vi "Main.vi"(8 "error in":errorcluster, 11 "Philosopher in":refnum<class "Philosopher.lvclass">) -> (0 "error out":errorcluster, 3 "Philosopher out":refnum<class "Philosopher.lvclass">)   [LabVIEW 2023, in "Philosopher.lvclass"]
uses:
  Philosopher.lvclass
  C:/Program Files (x86)/National Instruments/LabVIEW 2023/vi.lib/addons/_Workers/Library/Classes/Worker/Worker.lvclass
  Initialization Data.ctl
  <vilib>/addons/_Workers/Library/Classes/Message Queue/Message Queue.lvclass
  Philosopher.lvclass/Philosopher.ctl
  <vilib>/Utility/miscctls.llb/LVRectTypeDef.ctl
  <vilib>/addons/_Workers/Library/Classes/Message/Enqueue Message to Queue.vi
  <vilib>/addons/_Workers/Library/Classes/Message/Message.lvclass
  Table/Table.lvclass
  <vilib>/addons/_Workers/Library/Classes/Callback Message/Callback Message.lvclass
  Message Pump/Message Pump.lvclass
  <userlib>/_Workers/Worker Library/Message Pump/Workers/Message Pump/_Message Pump.lvclass
  C:/Program Files (x86)/National Instruments/LabVIEW 2023/vi.lib/addons/_Workers/Library/Classes/Workers Object/Workers Object.lvclass
  C:/Projects/DPP Workers/Workers/Philosopher/Philosopher.lvclass
panel:
  out "ID":i32
  out "State Picture":u16(ring)
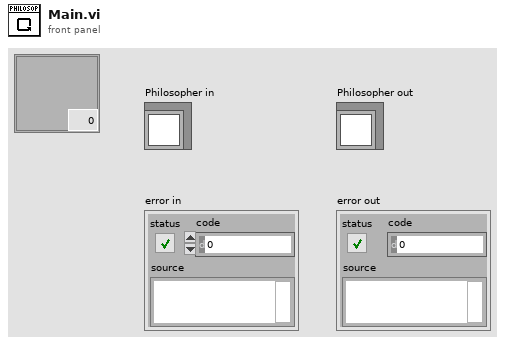
[diagram p1: front panel]
types:
  T1 = typedef "Philosopher.lvclass/Initialization Data.ctl" = cluster{"ID":i32, "MGQ Table":refnum<class "Message Queue.lvclass">}
  T2 = typedef "LVRectTypeDef.ctl" = cluster{"Left":i16, "Top":i16, "Right":i16, "Bottom":i16}
  T3 = typedef "Workers.lvlib/Case Label.ctl" = string
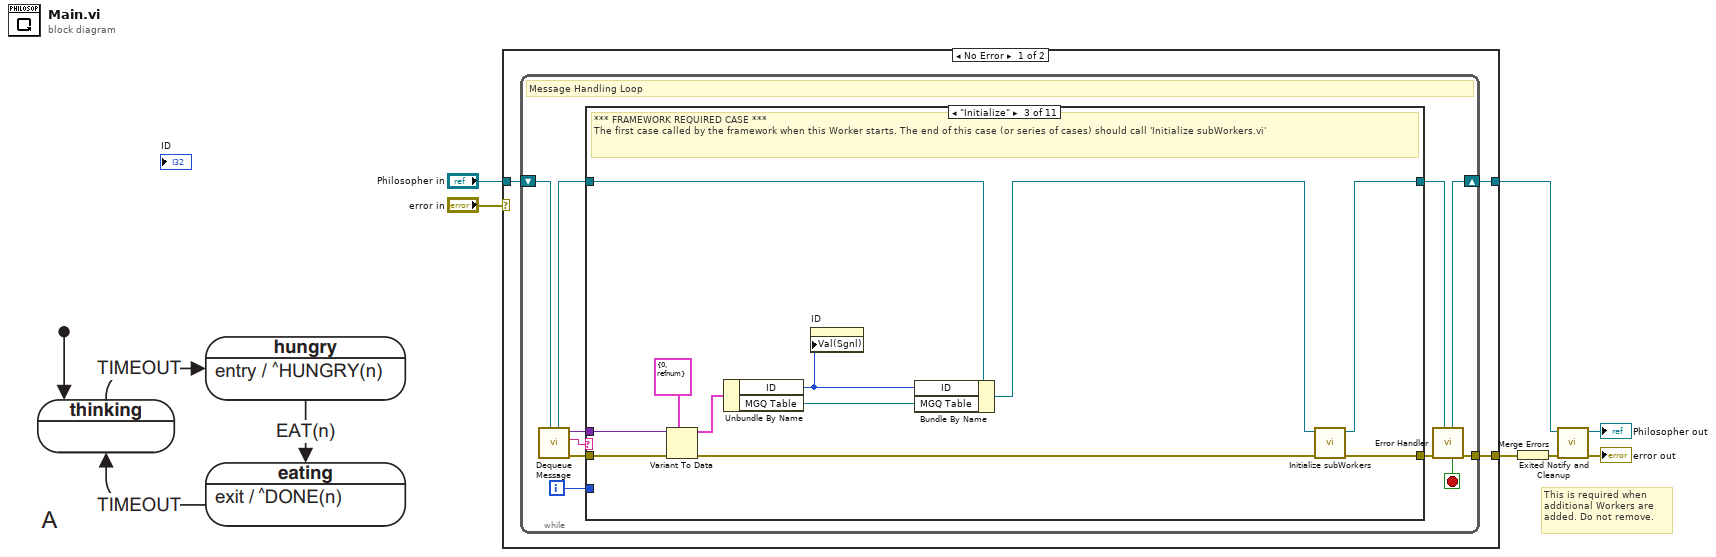
[diagram p0: block diagram]
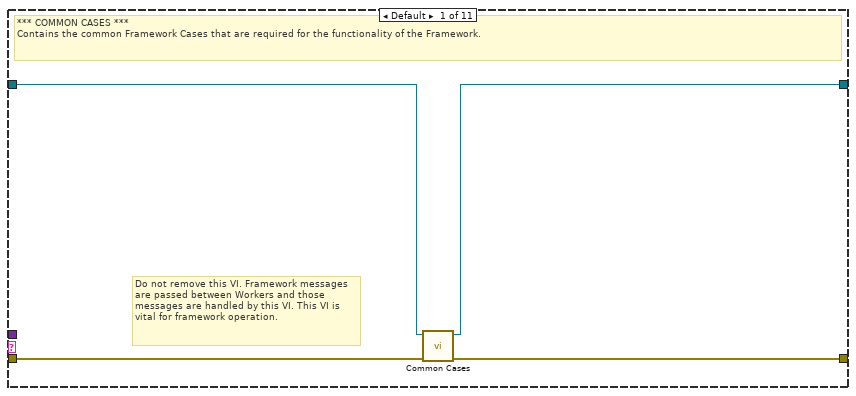
[diagram p2: hidden frame]
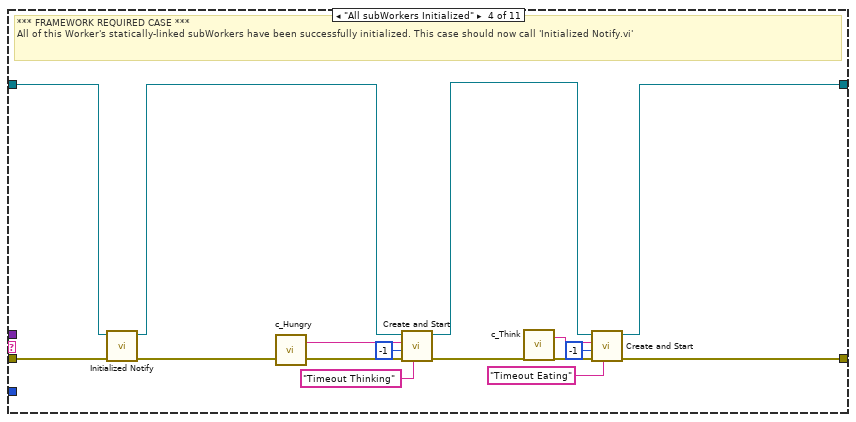
[diagram p4: hidden frame]
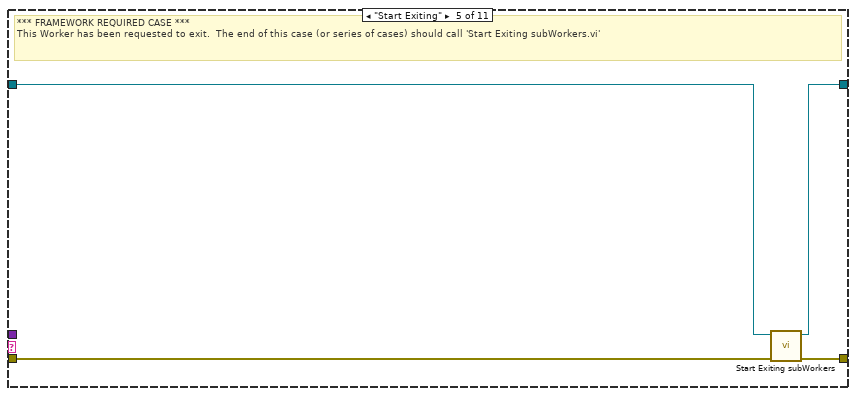
[diagram p5: hidden frame]
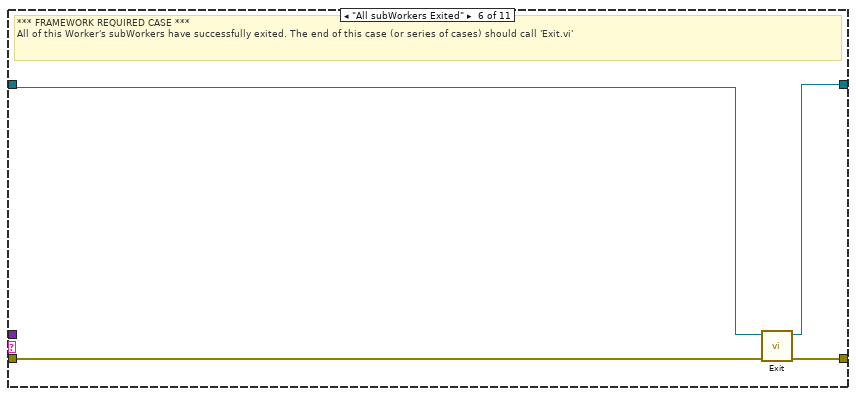
[diagram p6: hidden frame]
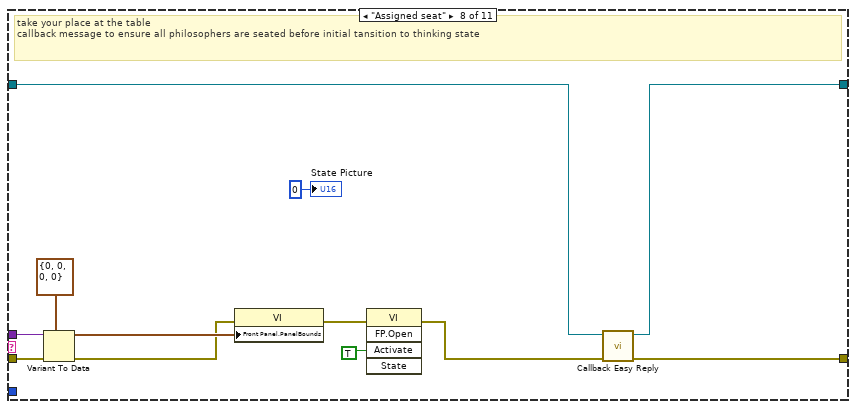
[diagram p8: hidden frame]
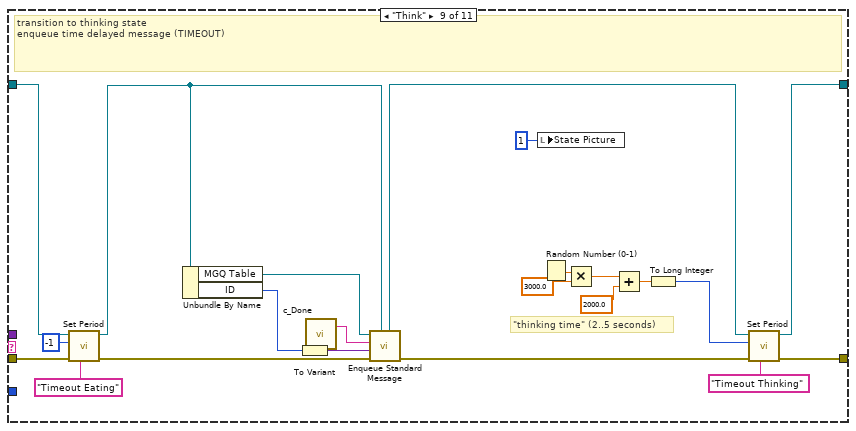
[diagram p9: hidden frame]
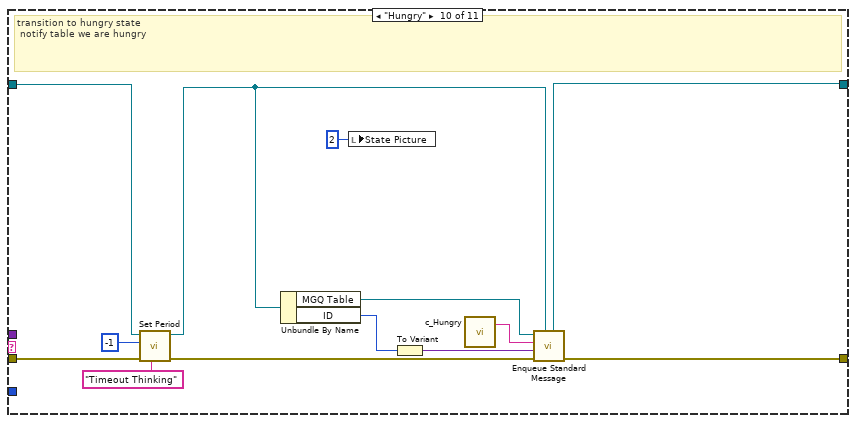
[diagram p10: hidden frame]
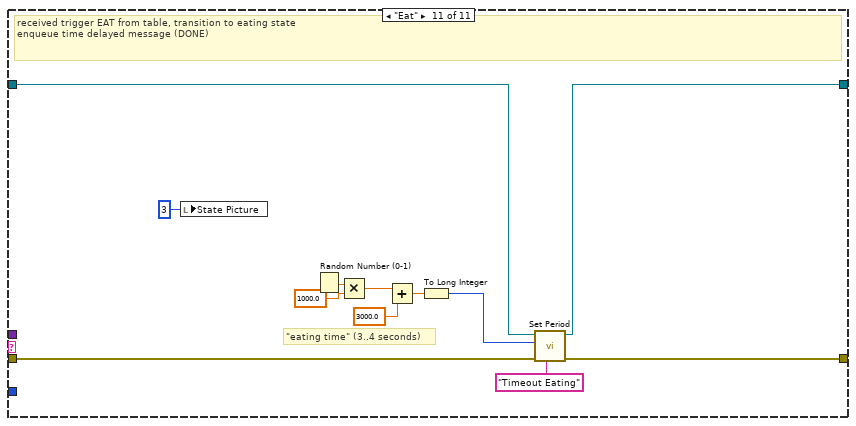
[diagram p11: hidden frame]
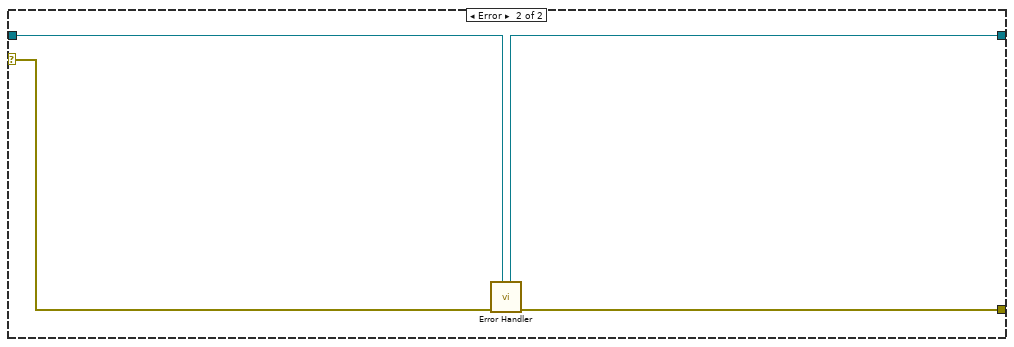
[diagram p12: hidden frame]
diagram:
  # "This is required when additional Workers are added. Do not remove."
  n1 = case shown="No Error" "error in" {
    tunnel: "Philosopher in" -> [w8 w123]
    tunnel: [w10 w124] -> w6
    tunnel: [w9 w122] -> w7
    selector: "error in" -> [_ w125]
    frame No Error {
      n2 = while {
        shift-right: [w19] -> w9
        shift-left: w8 -> [w21]
        tunnel: [w20] -> w10
        i -> [w11]
        stop <- w12 stop-if-true
        # "Message Handling Loop"
        n3 = call-dynamic "Dequeue Message.vi"("Worker"=w21) -> ("error out"=w18:errorcluster, "Case out"=w13:string, "Data out"=w14:variant, "Worker out"=w16:refnum<class "Philosopher.lvclass">)  [unwired: 6 in, 1 out]
        n4 = case "Worker MHL Case Structure (DO NOT CHANGE LABEL NAME)" shown="\"Initialize\"" w13 {
          tunnel: w18 -> [w25 w26 w36 w52 w54 w60 w61 w74 w86 w102 w116]
          tunnel: [w24 w26 w38 w47 w56 w59 w61 w65 w90 w97 w110] -> w17
          tunnel: w16 -> [w23 w27 w32 w51 w53 w57 w62 w63 w79 w100 w115]
          tunnel: [w22 w27 w37 w39 w55 w58 w62 w64 w88 w107 w114] -> w15
          tunnel: w14 -> [_ _ w34 _ _ _ _ w73 _ _ _]
          tunnel: w11 -> [_ _ _ _ _ _ _ _ _ _ _]
          frame Default {
            # "Do not remove this VI. Framework messages are passed between Workers and those messages are handled by this VI. This VI is vital for framework operation."
            # "*** COMMON CASES ***\nContains the common Framework Cases that are required for the functionality of the Framework."
            n5 = call-dynamic "Common Cases.vi"("error in"=w25, "Worker in"=w23) -> ("error out"=w24:errorcluster, "Worker out"=w22:refnum<class "Philosopher.lvclass">)  [unwired: 8 in]
          }
          frame "------ FRAMEWORK REQUIRED CASES ------" {
            # "Start of Framework Required Cases"
          }
          frame "Initialize" {
            # "*** FRAMEWORK REQUIRED CASE ***\nThe first case called by the framework when this Worker starts. The end of this case (or series of cases) should call 'Initialize subWorkers.vi'"
            n6 = Variant To Data(error in=w36, type=T1 {"ID"=0, "MGQ Table"=refnum} ("Initialization Data"), Variant=w34) -> (data=w30:T1, error out=w35:errorcluster)
            n7 = Unbundle By Name(w30) -> ("ID"=w28:i32, "MGQ Table"=w29:refnum<class "Message Queue.lvclass">)
            n8 = property on="ID" class="DigNum (strict)"("Val(Sgnl)"=w28) -> ()  [unwired: 2 in, 2 out]
            n9 = Bundle By Name(cluster=w32, "ID"=w28, "MGQ Table"=w29) -> (w33:refnum<class "Philosopher.lvclass">)
            n10 = call-dynamic "Initialize subWorkers.vi"("error in"=w35, "Worker"=w33) -> ("error out"=w38:errorcluster, "dup Worker out"=w37:refnum<class "Philosopher.lvclass">)  [unwired: 8 in]
          }
          frame "All subWorkers Initialized" {
            # "*** FRAMEWORK REQUIRED CASE ***\nAll of this Worker's statically-linked subWorkers have been successfully initialized. This case should now call 'Initialized Notify.vi'"
            n11 = call-dynamic "Initialized Notify.vi"("error in"=w52, "Worker"=w51) -> ("error out"=w50:errorcluster, "dup Worker out"=w49:refnum<class "Philosopher.lvclass">)  [unwired: 8 in]
            n12 = call "c_Hungry.vi"() -> ("Case Label"=w43:T3)  [unwired: 1 in]
            n13 = call "Create and Start.vi"("Pump Name"="Timeout Thinking", "error in (no error)"=w50, "Period in ms (-1)"=-1, "Case Label"=w43, "Worker"=w49) -> ("error out"=w46:errorcluster, "Worker out"=w45:refnum<class "Philosopher.lvclass">)  [unwired: 5 in]
            n14 = call "c_Think.vi"() -> ("Case Label"=w42:T3)  [unwired: 1 in]
            n15 = call "Create and Start.vi"("Pump Name"="Timeout Eating", "error in (no error)"=w46, "Period in ms (-1)"=-1, "Case Label"=w42, "Worker"=w45) -> ("error out"=w47:errorcluster, "Worker out"=w39:refnum<class "Philosopher.lvclass">)  [unwired: 5 in]
          }
          frame "Start Exiting" {
            # "*** FRAMEWORK REQUIRED CASE ***\nThis Worker has been requested to exit.  The end of this case (or series of cases) should call 'Start Exiting subWorkers.vi'"
            n16 = call-dynamic "Start Exiting subWorkers.vi"("error_in"=w54, "Worker"=w53) -> ("error out"=w56:errorcluster, "dup Worker out"=w55:refnum<class "Philosopher.lvclass">)  [unwired: 8 in]
          }
          frame "All subWorkers Exited" {
            # "*** FRAMEWORK REQUIRED CASE ***\nAll of this Worker's subWorkers have successfully exited. The end of this case (or series of cases) should call 'Exit.vi'"
            n17 = call-dynamic "Exit.vi"("error_in"=w60, "Worker"=w57) -> ("error out"=w59:errorcluster, "dup Worker out"=w58:refnum<class "Philosopher.lvclass">)  [unwired: 8 in]
          }
          frame "-----------------------------------------------" {
            # "End of Framework Required Cases"
          }
          frame "Assigned seat" {
            # "take your place at the table\ncallback message to ensure all philosophers are seated before initial tansition to thinking state"
            n18 = Variant To Data(error in=w74, type=T2 {"Left"=0, "Top"=0, "Right"=0, "Bottom"=0} ("Front Panel Window:Window Bounds"), Variant=w73) -> (data=w69:T2, error out=w68:errorcluster)
            n19 = property on="Property Node" class="VI"(error in=w68, "Front Panel.PanelBounds"=w69) -> (error out=w70:errorcluster)  [unwired: 1 in, 1 out]
            n20 = invoke on="Invoke Node" class="VI" method="FP.Open"(error in=w70, "Activate"=TRUE ("Activate?")) -> (error out=w66:errorcluster)  [unwired: 3 in, 4 out]
            n21 = call <vilib>:"Callback Easy Reply.vi"("error in"=w66, "Worker"=w63) -> ("error out"=w65:errorcluster, "dup Worker out"=w64:refnum<class "Philosopher.lvclass">)  [unwired: 8 in]
            "State Picture" <- u16 0 ("State Picture")
          }
          frame "Think" {
            # "\"thinking time\" (2..5 seconds)"
            # "transition to thinking state\nenqueue time delayed message (TIMEOUT)"
            n22 = call <userlib>:"Set Period.vi"("Pump Name"="Timeout Eating", "error in"=w86, "Period in ms (-1)"=-1, "Worker"=w79) -> ("error out"=w80:errorcluster, "Worker out"=w77:refnum<class "Philosopher.lvclass">)  [unwired: 6 in]
            n23 = Unbundle By Name(w77) -> ("MGQ Table"=w83:refnum<class "Message Queue.lvclass">, "ID"=w84:i32)
            n24 = To Variant(anything=w84) -> (Variant=w81:variant)
            n25 = call "c_Done.vi"() -> ("Case Label"=w82:T3)  [unwired: 1 in]
            n26 = call-poly <vilib>:"Enqueue Standard Message.vi"("Worker"=w77, "error in"=w80, "Data"=w81, "Case Label"=w82, "Message Queue"=w83) -> ("error out"=w75:errorcluster, "dup Worker out"=w78:refnum<class "Philosopher.lvclass">)  [unwired: 4 in, 1 out]
            n27 = local write "State Picture"(u16 1 ("State Picture")) -> ()
            n28 = Random Number (0-1)() -> (number: 0 to 1=w94:dbl)
            n29 = Multiply(x=w94, y=3000.0) -> (x*y=w95:dbl)
            n30 = Add(x=w95, y=2000.0) -> (x+y=w93:dbl)
            n31 = To Long Integer(number=w93) -> (32bit integer=w89:i32)
            n32 = call <userlib>:"Set Period.vi"("Pump Name"="Timeout Thinking", "error in"=w75, "Period in ms (-1)"=w89, "Worker"=w78) -> ("error out"=w90:errorcluster, "Worker out"=w88:refnum<class "Philosopher.lvclass">)  [unwired: 6 in]
          }
          frame "Hungry" {
            # "transition to hungry state\n notify table we are hungry"
            n33 = call <userlib>:"Set Period.vi"("Pump Name"="Timeout Thinking", "error in"=w102, "Period in ms (-1)"=-1, "Worker"=w100) -> ("error out"=w103:errorcluster, "Worker out"=w101:refnum<class "Philosopher.lvclass">)  [unwired: 6 in]
            n34 = Unbundle By Name(w101) -> ("MGQ Table"=w108:refnum<class "Message Queue.lvclass">, "ID"=w106:i32)
            n35 = local write "State Picture"(u16 2 ("State Picture")) -> ()
            n36 = To Variant(anything=w106) -> (Variant=w104:variant)
            n37 = call "c_Hungry.vi"() -> ("Case Label"=w105:T3)  [unwired: 1 in]
            n38 = call-poly <vilib>:"Enqueue Standard Message.vi"("Worker"=w101, "error in"=w103, "Data"=w104, "Case Label"=w105, "Message Queue"=w108) -> ("error out"=w97:errorcluster, "dup Worker out"=w107:refnum<class "Philosopher.lvclass">)  [unwired: 4 in, 1 out]
          }
          frame "Eat" {
            # "\"eating time\" (3..4 seconds)"
            # "received trigger EAT from table, transition to eating state\nenqueue time delayed message (DONE)"
            n39 = local write "State Picture"(u16 3 ("State Picture")) -> ()
            n40 = Random Number (0-1)() -> (number: 0 to 1=w120:dbl)
            n41 = Multiply(x=w120, y=1000.0) -> (x*y=w121:dbl)
            n42 = Add(x=w121, y=3000.0) -> (x+y=w112:dbl)
            n43 = To Long Integer(number=w112) -> (32bit integer=w111:i32)
            n44 = call <userlib>:"Set Period.vi"("Pump Name"="Timeout Eating", "error in"=w116, "Period in ms (-1)"=w111, "Worker"=w115) -> ("error out"=w110:errorcluster, "Worker out"=w114:refnum<class "Philosopher.lvclass">)  [unwired: 6 in]
          }
        }
        n45 = call-dynamic "Error Handler.vi"("Worker"=w15, "error_in"=w17) -> ("error out"=w20:errorcluster, "Stop Loop"=w12:bool, "Worker out"=w19:refnum<class "Philosopher.lvclass">)  [unwired: 7 in]
      }
    }
    frame Error {
      n46 = call-dynamic "Error Handler.vi"("Worker"=w123, "error_in"=w125) -> ("error out"=w124:errorcluster, "Worker out"=w122:refnum<class "Philosopher.lvclass">)  [unwired: 7 in, 1 out]
    }
  }
  n47 = Merge Errors(w6) -> (w3:errorcluster)
  n48 = call-dynamic "Exited Notify and Cleanup.vi"("error_in"=w3, "Worker"=w7) -> ("error out"=→"error out":errorcluster, "dup Worker out"=→"Philosopher out":refnum<class "Philosopher.lvclass">)  [unwired: 8 in]
